vi "Close Text File.vi"(8 "error in (no error)":errorcluster, 11 "Data Cluster":T1) -> (0 "error out":errorcluster, 3 "Status":string)   [LabVIEW 2020, in "Logging - Text.lvlib"]
uses:
  Logging - Text.lvlib
  Module Data--cluster.ctl
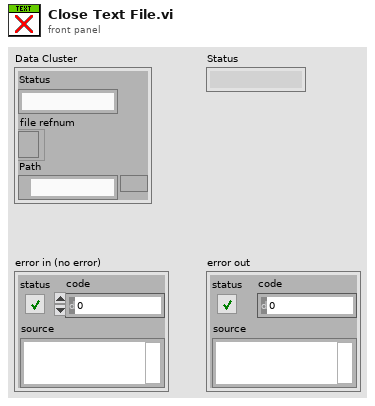
[diagram p1: front panel]
types:
  T1 = typedef "Logging - Text.lvlib/Module Data--cluster.ctl" = cluster{"Status":string, "file refnum":refnum<file>, "Path":path}
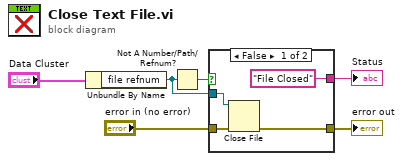
[diagram p0: block diagram]
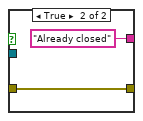
[diagram p2: hidden frame]
diagram:
  n1 = Unbundle By Name("Data Cluster") -> ("file refnum"=w4:refnum<file>)
  n2 = Not A Number/Path/Refnum?(number/path/refnum=w4) -> (NaN/Path/Refnum?=w5:bool)
  n3 = case shown="False" w5 {
    tunnel: "error in (no error)" -> [w10 w11]
    tunnel: [w9 w11] -> w3
    tunnel: w4 -> [w8 _]
    tunnel: ["File Closed" ("Status") "Already closed" ("Status")] -> w6
    frame False {
      n4 = Close File(refnum=w8, error in=w10) -> (error out=w9:errorcluster)  [unwired: 1 out]
    }
    frame True {
    }
  }
  "Status" <- w6
  "error out" <- w3
